vi "EXTRACT-DATA-DBL.vi"(2 "DBL":dbl, 7 "Data":u8[](array[numeric])) -> (4 "Value":dbl, 8 "Min":dbl, 10 "Max":dbl, 15 "Inc":dbl)   [LabVIEW 2019]
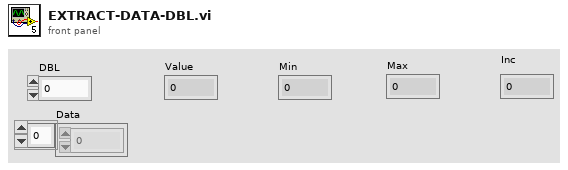
[diagram p1: front panel]
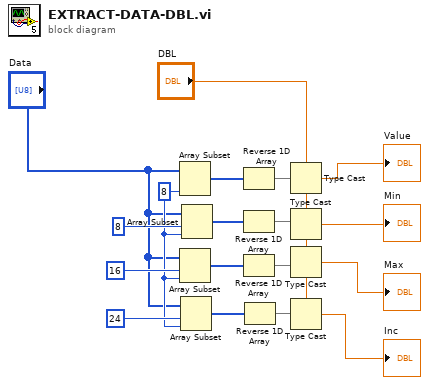
[diagram p0: block diagram]
diagram:
  w12 = 8 ("length")
  n1 = Array Subset(array="Data", length=w12) -> (w16:u8[])  [unwired: 1 in]
  n2 = Array Subset(array="Data", index=16, length=w12) -> (w17:u8[])
  n3 = Array Subset(array="Data", index=24, length=w12) -> (w11:u8[])
  n4 = Array Subset(array="Data", index=8, length=w12) -> (w18:u8[])
  n5 = Reverse 1D Array(array=w16) -> (reversed array=w10:u8[])
  n6 = Reverse 1D Array(array=w18) -> (reversed array=w9:u8[])
  n7 = Reverse 1D Array(array=w17) -> (reversed array=w8:u8[])
  n8 = Reverse 1D Array(array=w11) -> (reversed array=w7:u8[])
  n9 = Type Cast(type="DBL", x=w10) -> (*(type *) &x=→"Value":dbl)
  n10 = Type Cast(type="DBL", x=w9) -> (*(type *) &x=→"Min":dbl)
  n11 = Type Cast(type="DBL", x=w8) -> (*(type *) &x=→"Max":dbl)
  n12 = Type Cast(type="DBL", x=w7) -> (*(type *) &x=→"Inc":dbl)
